vi "TB-Config.vi"(0 "Params":T6={"Low cutoff (kHz)"=0.0, "High cutoff (kHz)"=0.0, "Duration (min)"=0.0, "dB SPL"=0.0, "Waveform"=enum."Noise", "WAVfile"=path "", "refWav"=path "", "use mic correction"=FALSE, "micCorrFile"=path "", "Pistonphone Level (dB SPL)"=0.0, "Sampling rate (Hz)"=0.0, "Buffer length (s)"=0.0, "Stream mic"=FALSE, "Fine adjust"={"Max"=0.0, "Min"=0.0}, "Mic gain"=0.0, "atten"=0.0, "Allow Slack"=FALSE, "max starts"=0, "Freq (kHz)"=8.0, "Tma (s)"=0.0, "Streamed"=[], "Drive"="", "Speaker"="", "Mic"="", "Analysis"={"Method"=enum."Default", "resol (Hz)"=0.0, "nfreq"=0, "signal"=""}}, 1 "Exposure?":bool, 9 "ID":string, 11 "error in (no error)":errorcluster, 12 "Fine adjust (dB)":dbl) -> (4 "state":T3, 10 "Num Buffers":i32, 13 "stimulus state":T1, 15 "error out":errorcluster)   [LabVIEW 2020]
uses:
  Typedefs/TB-Parameters.ctl
  Typedefs/TB-Analysis Parameters.ctl
  epl-vi-lib/Signal Synthesis VIs/4th Generation/Classes/SignalManager/SignalManager.lvclass
  Typedefs/TB-Runtime state.ctl
  <vilib>/sound2/lvsound2.llb/Sound File Refnum.ctl
  Typedefs/TB-Setup Log.ctl
  Typedefs/TB-Analysis State.ctl
  Typedefs/TB-Stimulus State.ctl
  09a94c86-6c43-4da1-a84f-5805afaf77f7.vi
  56413d8f-21dc-4b54-979e-3d43055f554d.vi
  epl-vi-lib/PXI DAQ VIs/AIDI/AIDI-Engine.vi
  epl-vi-lib/PXI DAQ VIs/AODO/AODO-Engine.vi
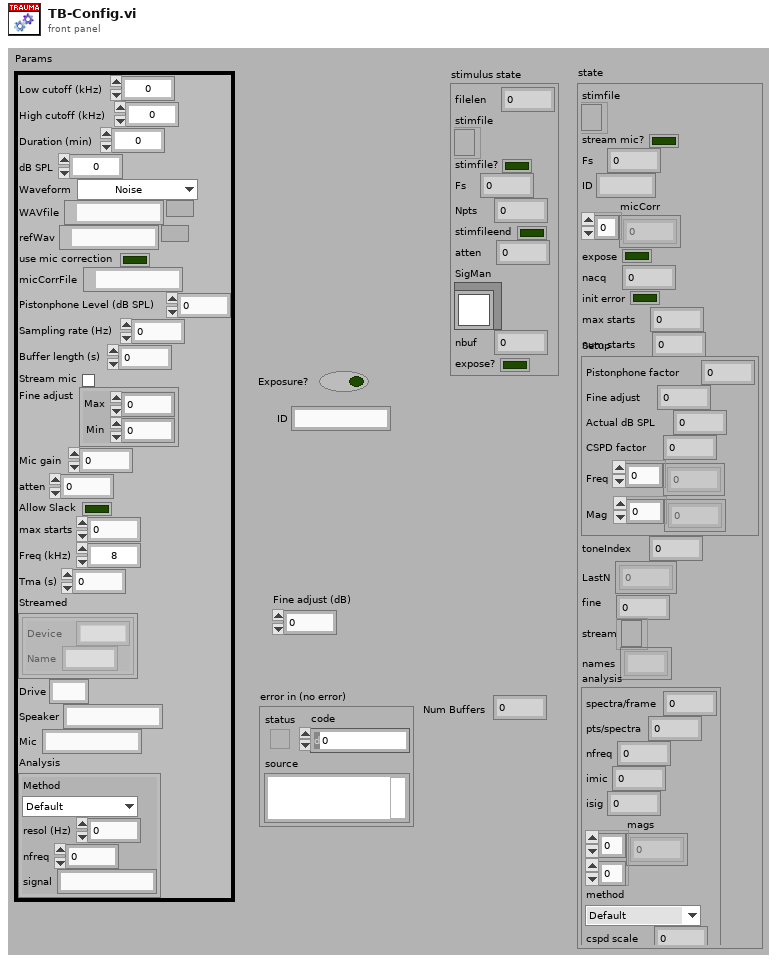
[diagram p1: front panel]
types:
  T1 = typedef "TB-Stimulus State.ctl" = cluster{"filelen":i32, "stimfile":T2, "stimfile?":bool, "Fs":dbl, "Npts":i32, "stimfileend":bool, "atten":dbl, "SigMan":refnum<class "SignalManager.lvclass">, "nbuf":i32, "expose?":bool}
  T2 = typedef "Sound File Refnum.ctl" = refnum<file>
  T3 = typedef "TB-Runtime state.ctl" = cluster{"stimfile":T2, "stream mic?":bool, "Fs":dbl, "ID":string, "micCorr":dbl[], "expose":bool, "nacq":i32, "init error":bool, "max starts":i32, "num starts":i32, "Setup":T4, "toneIndex":i32, "LastN":dbl[], "fine":dbl, "stream":refnum<file>, "names":string[], "analysis":T5}
  T4 = typedef "TB-Setup Log.ctl" = cluster{"Pistonphone factor":dbl, "Fine adjust":dbl, "Actual dB SPL":dbl, "CSPD factor":dbl, "Freq":dbl[], "Mag":dbl[]}
  T5 = typedef "TB-Analysis State.ctl" = cluster{"spectra/frame":i32, "pts/spectra":i32, "nfreq":i32, "imic":i32, "isig":i32, "mags":dbl[][], "method":enum16{"Default", "Periodogram", "Cross-spectrum"}, "cspd scale":dbl}
  T6 = typedef "TB-Parameters.ctl" = cluster{"Low cutoff (kHz)":dbl, "High cutoff (kHz)":dbl, "Duration (min)":dbl, "dB SPL":dbl, "Waveform":enum16{"Noise", "File", "Tone"}, "WAVfile":path, "refWav":path, "use mic correction":bool, "micCorrFile":path, "Pistonphone Level (dB SPL)":dbl, "Sampling rate (Hz)":dbl, "Buffer length (s)":dbl, "Stream mic":bool, "Fine adjust":cluster{"Max":dbl, "Min":dbl}, "Mic gain":dbl, "atten":dbl, "Allow Slack":bool, "max starts":i32, "Freq (kHz)":dbl, "Tma (s)":dbl, "Streamed":cluster{"Device":string, "Name":string}[], "Drive":string, "Speaker":string, "Mic":string, "Analysis":T7}
  T7 = typedef "TB-Analysis Parameters.ctl" = cluster{"Method":enum16{"Default", "Periodogram", "Cross-spectrum"}, "resol (Hz)":dbl, "nfreq":i32, "signal":string}
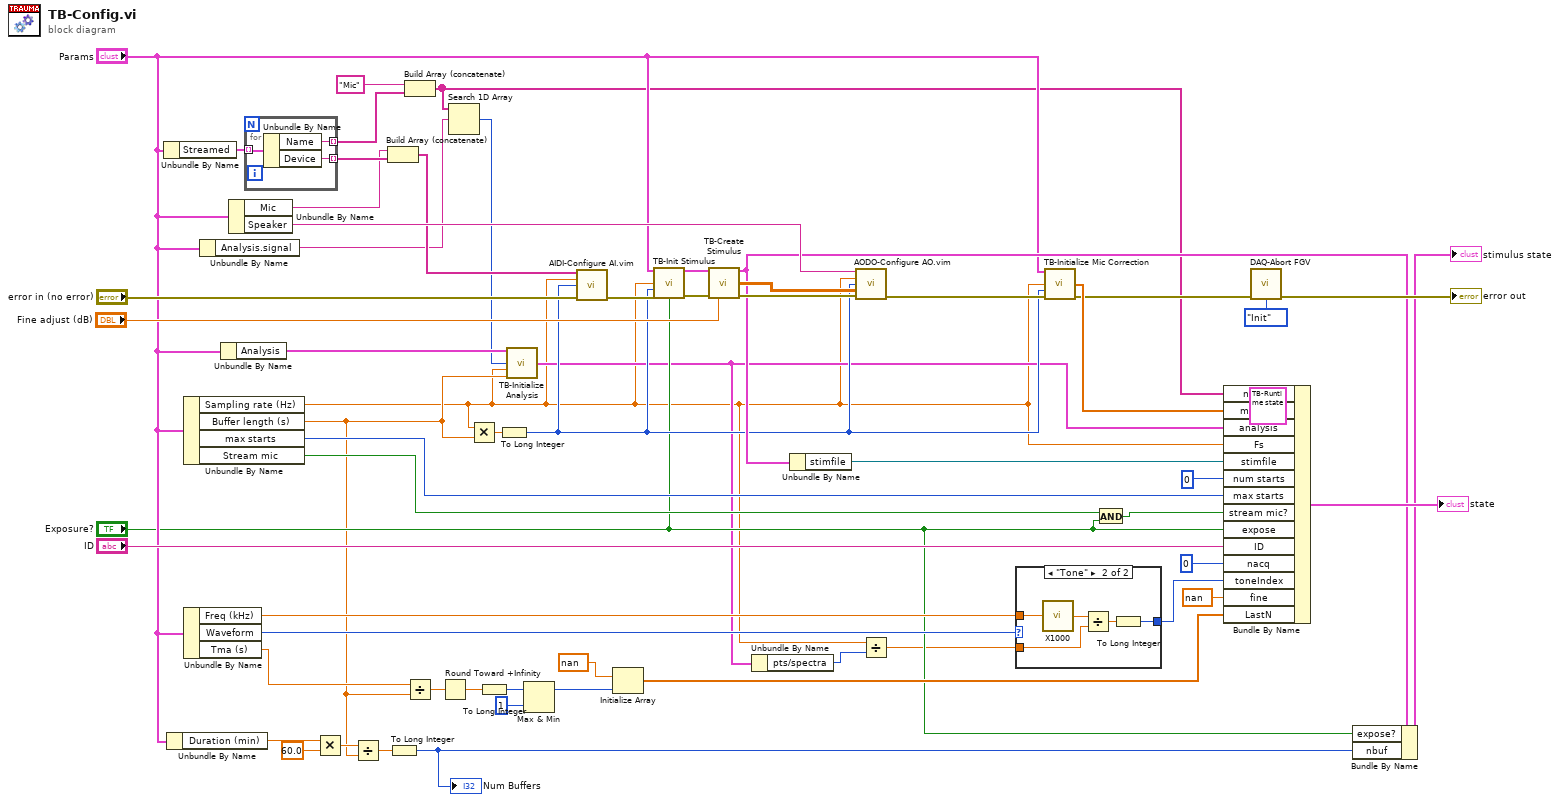
[diagram p0: block diagram]
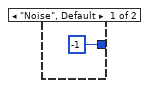
[diagram p2: hidden frame]
diagram:
  n1 = Unbundle By Name("Params") -> ("Streamed"=w34:cluster{"Device":string, "Name":string}[])
  n2 = Unbundle By Name("Params") -> ("Duration (min)"=w59:dbl)
  n3 = Unbundle By Name("Params") -> ("Sampling rate (Hz)"=w1:dbl, "Buffer length (s)"=w4:dbl, "max starts"=w51:i32, "Stream mic"=w52:bool)
  n4 = Unbundle By Name("Params") -> ("Freq (kHz)"=w44:dbl, "Waveform"=w46:enum16{"Noise", "File", "Tone"}, "Tma (s)"=w43:dbl)
  n5 = Unbundle By Name("Params") -> ("Analysis.signal"=w8:string)
  n6 = Unbundle By Name("Params") -> ("Analysis"=w12:T7)
  n7 = Unbundle By Name("Params") -> ("Mic"=w27:string, "Speaker"=w28:string)
  n8 = for {
    tunnel: w34 -> [w63] mode=indexing
    tunnel: [w62] -> w30 mode=indexing
    tunnel: [w61] -> w33 mode=indexing
    n9 = Unbundle By Name(w63) -> ("Name"=w61:string, "Device"=w62:string)
  }
  n10 = Multiply(x=w59, y=60.0) -> (x*y=w57:dbl)
  n11 = Divide(x=w57, y=w4) -> (x/y=w56:dbl)
  n12 = Build Array (concatenate)(w27, w30) -> (w11:string[])
  n13 = To Long Integer(number=w56) -> (32bit integer=w13:i32)
  "Num Buffers" <- w13
  n14 = Build Array (concatenate)("Mic", w33) -> (w9:string[])
  n15 = Divide(x=w43, y=w4) -> (x/y=w42:dbl)
  n16 = Round Toward +Infinity(x=w42) -> (ceil(x): smallest int >= x=w41:dbl)
  n17 = Search 1D Array(1D array=w9, element=w8) -> (index of element=w7:i32)  [unwired: 1 in]
  n18 = Multiply(x=w1, y=w4) -> (x*y=w60:dbl)
  n19 = To Long Integer(number=w41) -> (32bit integer=w40:i32)
  n20 = To Long Integer(number=w60) -> (32bit integer=w15:i32)
  n21 = call "TB-Initialize Analysis.vi"("Analysis"=w12, "isig"=w7, "Fs (Hz)"=w1, "Buffer length (s)"=w4) -> ("state"=w5:T5)  [unwired: 11 in]
  n22 = Max & Min(x=w40, y=1) -> (max(x,y)=w36:i32)  [unwired: 1 out]
  n23 = call "AIDI-Configure AI.vim"("AI.Channels"=w11, "AI.Fs (Hz)"=w1, "AI.Npts"=w15, "error in (no error)"="error in (no error)") -> ("error out"=w23:errorcluster)  [unwired: 11 in]
  n24 = Initialize Array(nan, w36) -> (w38:dbl[])
  n25 = call "TB-Init Stimulus.vi"("Exposure parameters"="Params", "Sampling rate (Hz)"=w1, "Npts"=w15, "error in (no error)"=w23, "Exposure"="Exposure?") -> ("state"=w20:T1, "error out"=w21:errorcluster)  [unwired: 9 in]
  n26 = call "TB-Create Stimulus.vi"("state"=w20, "error in (no error)"=w21, "Fine adjust (dB)"="Fine adjust (dB)") -> ("state out"=w16:T1, "Stimulus"=w18:dbl[][], "error out"=w17:errorcluster)  [unwired: 9 in, 1 out]
  n27 = Unbundle By Name(w5) -> ("pts/spectra"=w3:i32)
  n28 = Unbundle By Name(w16) -> ("stimfile"=w47:T2)
  n29 = call "AODO-Configure AO.vim"("AO.Channels"=w28, "AO.Fs (Hz)"=w1, "AO.Npts"=w15, "AO"=w18, "error in (no error)"=w17) -> ("error out"=w22:errorcluster)  [unwired: 10 in]
  n30 = Divide(x=w1, y=w3) -> (x/y=w2:dbl)
  n31 = case shown="\"Tone\"" w46 {
    tunnel: [-1 w65] -> w45
    tunnel: w2 -> [_ w67]
    tunnel: w44 -> [_ w69]
    frame "Noise", Default {
    }
    frame "Tone" {
      n32 = call "X1000.vi"("X"=w69) -> ("X/1000"=w68:dbl)
      n33 = Divide(x=w68, y=w67) -> (x/y=w66:dbl)
      n34 = To Long Integer(number=w66) -> (32bit integer=w65:i32)
    }
  }
  n35 = call "TB-Initialize Mic Correction.vi"("Exposure parameters"="Params", "Sampling rate (Hz)"=w1, "Npts"=w15, "error in (no error)"=w22) -> ("micCorr"=w49:dbl[], "error out"=w25:errorcluster)  [unwired: 10 in]
  n36 = And(x=w52, y="Exposure?") -> (x .and. y?=w31:bool)
  n37 = Bundle By Name(cluster=T3 {"stimfile"=refnum, "stream mic?"=FALSE, "Fs"=0.0, "ID"="", "micCorr"=[], "expose"=FALSE, "nacq"=0, "init error"=FALSE, "max starts"=0, "num starts"=0, "Setup"={"Pistonphone factor"=0.0, "Fine adjust"=0.0, "Actual dB SPL"=0.0, "CSPD factor"=0.0, "Freq"=[], "Mag"=[]}, "toneIndex"=0, "LastN"=[], "fine"=0.0, "stream"=refnum, "names"=[], "analysis"={"spectra/frame"=0, "pts/spectra"=0, "nfreq"=0, "imic"=0, "isig"=0, "mags"=[], "method"=enum."Default", "cspd scale"=0.0}} ("state"), "names"=w9, "micCorr"=w49, "analysis"=w5, "Fs"=w1, "stimfile"=w47, "num starts"=0, "max starts"=w51, "stream mic?"=w31, "expose"="Exposure?", "ID"="ID", "nacq"=0 ("navg"), "toneIndex"=w45, "fine"=nan, "LastN"=w38) -> (→"state":T3)
  n38 = call "DAQ-Abort FGV.vi"("error in (no error)"=w25, "Action"=enum16{"Default", "Init", "Abort", "1st error"}."Init") -> ("Errors"=→"error out":errorcluster)  [unwired: 11 in, 2 out]
  n39 = Bundle By Name(cluster=w16, "expose?"="Exposure?", "nbuf"=w13) -> (→"stimulus state":T1)
